vi "Execute_Row.vi"(3 "Simulate/Run":T2, 5 "Traverse line":T3 {"Row Duration (mins)" format="%#.1f"; "Row No" min=0; "Trace Gas Concentration (%)" min=0.0 format="%#.2f"; "Emission Rate (l/min)" format="%#.2f"; "Tunnel Speed" format="%#.2f"; "Start X" format="%#.2f"; "Start Y" format="%#.2f"; "Start Z" format="%#.2f"; "End X" format="%#.2f"; "End Y" format="%#.2f"; "End Z" format="%#.2f"; "Averaging time (min)" min=0.0 format="%#.2f"}) -> (1 "Status":T1, 2 "Traverse line out":T3 {"Row Duration (mins)" format="%#.1f"; "Row No" min=0; "Trace Gas Concentration (%)" min=0.0 format="%#.2f"; "Emission Rate (l/min)" format="%#.2f"; "Tunnel Speed" format="%#.2f"; "Start X" format="%#.2f"; "Start Y" format="%#.2f"; "Start Z" format="%#.2f"; "End X" format="%#.2f"; "End Y" format="%#.2f"; "End Z" format="%#.2f"; "Averaging time (min)" min=0.0 format="%#.2f"})   [LabVIEW 2010]
uses:
  Traverse_cluster.ctl
  Spacing.ctl
  Controls/Multi_run_mode.ctl
  Controls/User_Specific_mode.ctl
  Multi_Run_Status.ctl
  Controls/Save_Data.ctl
  Controls/Setup.ctl
  Globals/Constants_global.vi
  Globals/Extra_Commands_Global.vi
  Globals/Trav_pos_global.vi
panel:
  # "X           Y            Z"
  # "Start"
  # "End"
  # "X           Y            Z"
  # "Start"
  # "End"
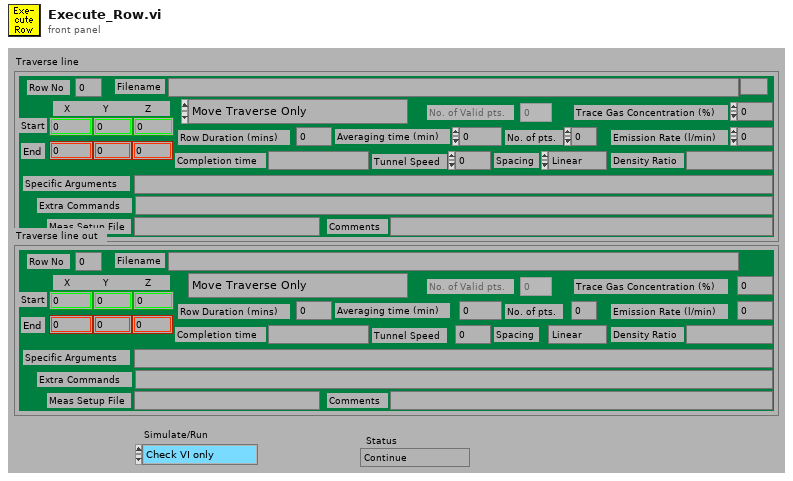
[diagram p1: front panel]
types:
  T1 = typedef "Multi_Run_Status.ctl" = enum16{"Continue", "Jump to Next Point", "Jump to Next Row", "Jump To Fall Back", "Terminate Run"}
  T2 = typedef "User_Specific_mode.ctl" = enum16{"Check VI only", "Run VI"}
  T3 = typedef "Traverse_cluster.ctl" = cluster{"Start X":dbl, "Start Y":dbl, "Start Z":dbl, "End X":dbl, "End Y":dbl, "End Z":dbl, "No. of pts.":i32, "Spacing":T4, "Filename":path, "Tunnel Speed":dbl, "Averaging time (min)":dbl, "Extra Commands":string, "Specific Arguments":string, "Emission Rate (l/min)":dbl, "Trace Gas Concentration (%)":dbl, "Density Ratio":string, "Comments":string, "Row No":i32, "Row Type Selector":T5, "Completion time":string, "Row Duration (mins)":dbl, "No. of Valid pts.":i32, "Meas Setup File":string}
  T4 = typedef "Spacing.ctl" = enum16{"Linear", "Log", "Gauss", "Specified", "N/A"}
  T5 = typedef "Multi_run_mode.ctl" = enum16{"Move Traverse Only", "Set Tunnel Speed Only", "Set Source Only", "Set Measurement Conditions", "Single Measurement", "Vertical Profile", "Lateral Profile", "Longitudinal Profile", "Explore Volume", "Multi-Axis Profile", "Auto Calibrate", "Meas Fast FID Bkgnd", "Check Beam Power", "Scanning Valve Measurement", "Run VI Named:", "Set ADAM Ch", "Wait (minutes)", "Send Message", "Synchronize With:", "Fall Back to this Row", "Turn Off Row Repeating", "Blank Row"}
  T6 = typedef "Save_Data.ctl" = enum16{"Save No Data", "Save Data"}
  T7 = typedef "Setup.ctl" = enum16{"Run Program", "Show Setup", "Save Current Setup", "Setup Front Panel"}
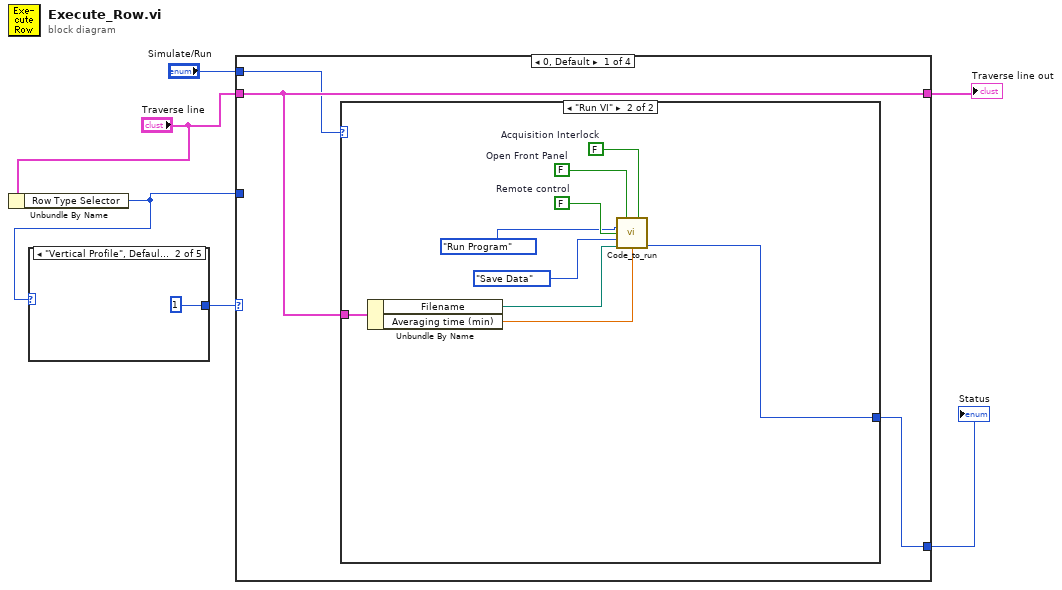
[diagram p0: block diagram]
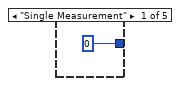
[diagram p2: hidden frame]
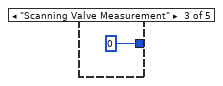
[diagram p3: hidden frame]
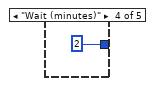
[diagram p4: hidden frame]
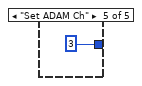
[diagram p5: hidden frame]
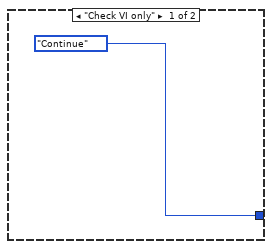
[diagram p6: hidden frame]
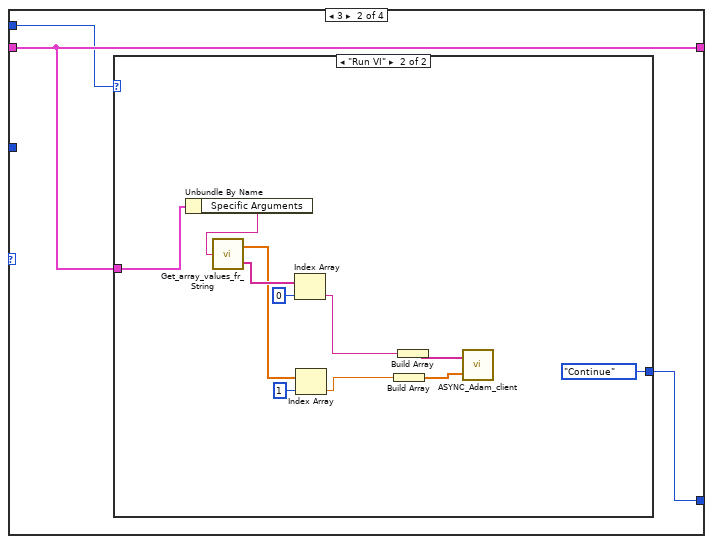
[diagram p7: hidden frame]
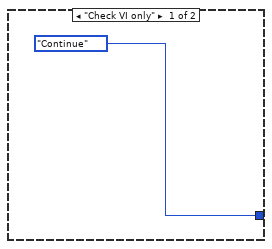
[diagram p8: hidden frame]
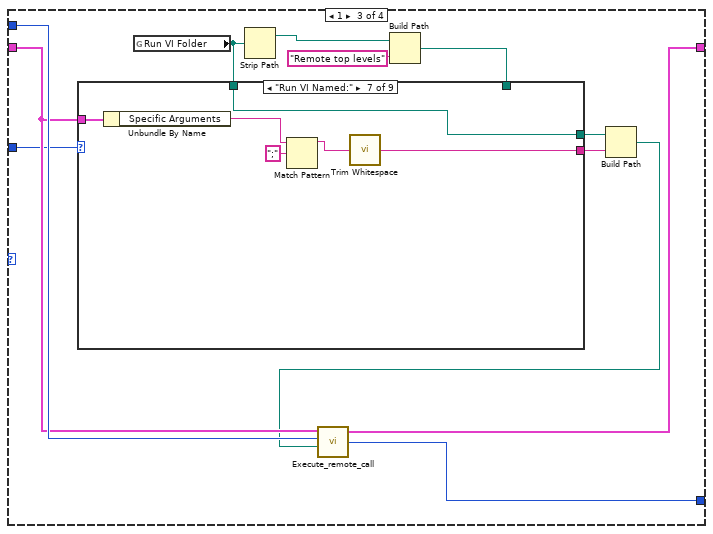
[diagram p9: hidden frame]
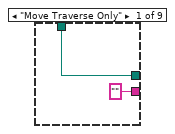
[diagram p10: hidden frame]
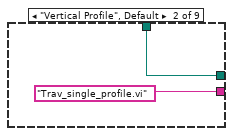
[diagram p11: hidden frame]
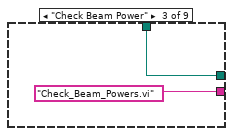
[diagram p12: hidden frame]
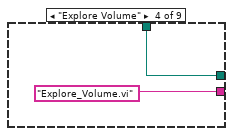
[diagram p13: hidden frame]
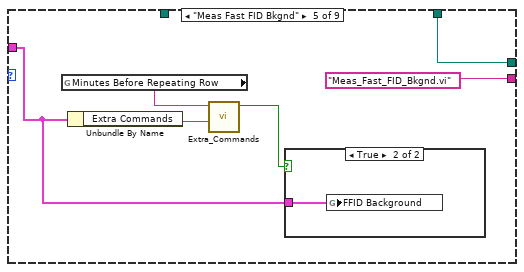
[diagram p14: hidden frame]
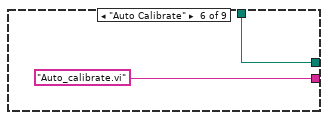
[diagram p16: hidden frame]
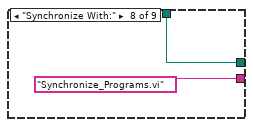
[diagram p17: hidden frame]
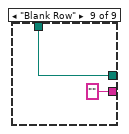
[diagram p18: hidden frame]
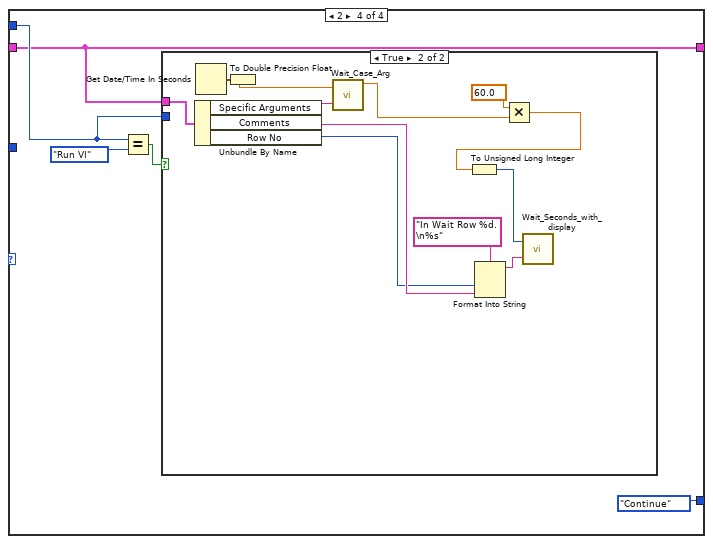
[diagram p19: hidden frame]
diagram:
  n1 = Unbundle By Name("Traverse line") -> ("Row Type Selector"=w2:T5)
  n2 = case shown="\"Vertical Profile\", Default" w2 {
    tunnel: [0 1 0 2 3] -> w3
    frame "Single Measurement" {
    }
    frame "Vertical Profile", Default {
    }
    frame "Scanning Valve Measurement" {
    }
    frame "Wait (minutes)" {
    }
    frame "Set ADAM Ch" {
    }
  }
  n3 = case shown="0, Default" w3 {
    tunnel: [w14 w27 w47 Multi_Run_Status."Continue" ("Status")] -> w1
    tunnel: "Traverse line" -> [w13 w26 w49 w80]
    tunnel: [w13 w26 w51 w80] -> w6
    tunnel: "Simulate/Run" -> [w12 w25 w50 w82]
    tunnel: w2 -> [_ _ w48 _]
    frame 0, Default {
      n4 = case shown="\"Run VI\"" w12 {
        tunnel: [Multi_Run_Status."Continue" ("Status") w24] -> w14
        tunnel: w13 -> [_ w23]
        frame "Check VI only" {
        }
        frame "Run VI" {
          w18 = FALSE  # Acquisition Interlock
          w19 = FALSE  # Open Front Panel
          w21 = FALSE  # Remote control
          n5 = Unbundle By Name(w23) -> ("Filename"=w22:path, "Averaging time (min)"=w20:dbl)
          n6 = call "Code_to_run.vi"("Open Front Panel"=w19, "Acquisition Interlock"=w18, "setup"=Setup."Run Program", "Remote control"=w21, "File"=Save_Data."Save Data", "Results Filename"=w22, "Averaging time (min)"=w20) -> ("Status"=w24:T1)  [unwired: 4 in, 4 out]
        }
      }
    }
    frame 3 {
      n7 = case shown="\"Run VI\"" w25 {
        tunnel: [Multi_Run_Status."Continue" ("Status") Multi_Run_Status."Continue" ("Status")] -> w27
        tunnel: w26 -> [_ w34]
        frame "Check VI only" {
        }
        frame "Run VI" {
          n8 = Unbundle By Name(w34) -> ("Specific Arguments"=w33:string)
          n9 = call "Get_array_values_fr_String.vi"("String Value"=w33) -> ("Numeric Array"=w31:dbl[], "String array"=w36:string[])
          n10 = Index Array(array=w36, index=0) -> (element=w35:string)
          n11 = Index Array(array=w31, index=1) -> (element=w30:dbl)
          n12 = Build Array(w30) -> (w38:dbl[])
          n13 = Build Array(w35) -> (w39:string[])
          n14 = call "ASYNC_Adam_client.vi"("Values"=w38, "Channel Names"=w39) -> ()  [unwired: 2 out]
        }
      }
    }
    frame 1 {
      n15 = global read "Constants_global.vi" "Run VI Folder"() -> (w40:path)
      n16 = Strip Path(path=w40) -> (stripped path=w41:path)  [unwired: 1 out]
      n17 = Build Path(base path=w41, name or relative path="Remote top levels") -> (appended path=w45:path)
      n18 = case shown="\"Run VI Named:\"" w48 {
        tunnel: w45 -> [w53 w55 w57 w59 w65 w68 _ w76 w78]
        tunnel: w49 -> [_ _ _ _ w60 _ w74 _ _]
        tunnel: [w53 w55 w57 w59 w65 w68 w73 w76 w78] -> w44
        tunnel: ["" ("name") "Trav_single_profile.vi" "Check_Beam_Powers.vi" "Explore_Volume.vi" "Meas_Fast_FID_Bkgnd.vi" "Auto_calibrate.vi" w69 "Synchronize_Programs.vi" "" ("name")] -> w43
        tunnel: w40 -> [_ _ _ _ _ _ w73 _ _]
        frame "Move Traverse Only" {
        }
        frame "Vertical Profile", Default {
        }
        frame "Check Beam Power" {
        }
        frame "Explore Volume" {
        }
        frame "Meas Fast FID Bkgnd" {
          n19 = global read "Extra_Commands_Global.vi" "Minutes Before Repeating Row"() -> (w63:string)
          n20 = Unbundle By Name(w60) -> ("Extra Commands"=w62:string)
          n21 = call "Extra_Commands.vi"("String to Search"=w62, "Command"=w63) -> ("Command Found"=w61:bool)  [unwired: 1 in, 4 out]
          n22 = case shown="True" w61 {
            tunnel: w60 -> [_ w66]
            frame False {
            }
            frame True {
              n23 = global write "Trav_pos_global.vi" "FFID Background"(w66) -> ()
            }
          }
        }
        frame "Auto Calibrate" {
        }
        frame "Run VI Named:" {
          n24 = Unbundle By Name(w74) -> ("Specific Arguments"=w71:string)
          n25 = Match Pattern(string=w71, regular expression=";") -> (before substring=w70:string)  [unwired: 4 out]
          n26 = call <vilib>:"Trim Whitespace.vi"("string"=w70) -> ("trimmed string"=w69:string)  [unwired: 1 in]
        }
        frame "Synchronize With:" {
        }
        frame "Blank Row" {
        }
      }
      n27 = Build Path(base path=w44, name or relative path=w43) -> (appended path=w42:path)
      n28 = call "Execute_remote_call.vi"("Traverse line"=w49, "Simulate/Run"=w50, "VI to run"=w42) -> ("Traverse Out"=w51:T3, "Status"=w47:T1)  [unwired: 1 in, 3 out]
    }
    frame 2 {
      n29 = Equal?(x=w82, y=User_Specific_mode."Run VI" ("Simulate/Run")) -> (x = y?=w81:bool)
      n30 = case shown="True" w81 {
        tunnel: w80 -> [_ w89]
        tunnel: w82 -> [_ _]
        frame False {
        }
        frame True {
          n31 = Unbundle By Name(w89) -> ("Specific Arguments"=w90:string, "Comments"=w85:string, "Row No"=w84:i32)
          n32 = Get Date/Time In Seconds() -> (seconds since 1Jan1904=w88:timestamp)
          n33 = To Double Precision Float(number=w88) -> (double precision float=w91:dbl)
          n34 = call "Wait_Case_Arg.vi"("Specific Argument"=w90, "seconds since 1Jan1904"=w91) -> ("Minutes To Wait"=w92:dbl)  [unwired: 4 out]
          n35 = Format Into String(format string="In Wait Row %d.\n%s", w84, w85) -> (resulting string=w87:string)  [unwired: 2 in, 1 out]
          n36 = Multiply(x=60.0, y=w92) -> (x*y=w93:dbl)
          n37 = To Unsigned Long Integer(number=w93) -> (unsigned 32bit integer=w94:u32)
          n38 = call "Wait_Seconds_with_display.vi"("Message"=w87, "Seconds to wait"=w94) -> ()  [unwired: 2 out]
        }
      }
    }
  }
  "Traverse line out" <- w6
  "Status" <- w1
